vi "Write EEPROM User Area.vi"(8 "error in (no error)":errorcluster, 10 "User Area Data":u8[](array[numeric]) format="%x", 11 "Handle":u64) -> (0 "error out":errorcluster, 3 "Handle out":u64)   [LabVIEW 2019, in "D2XX-lv.lvlib"]
doc: "Write data into the EEPROM user area."
uses:
  D2XX-lv.lvlib
  <instrlib>/_D2XX/D2XX/D2XX.lvlib
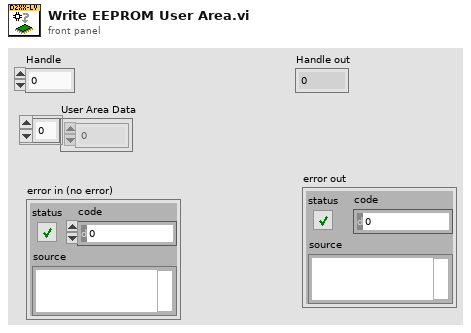
[diagram p1: front panel]
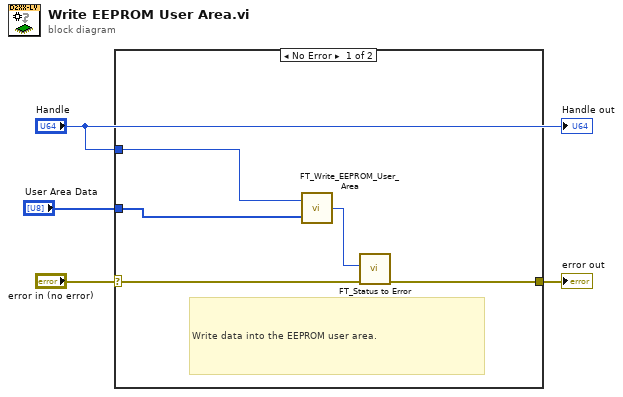
[diagram p0: block diagram]
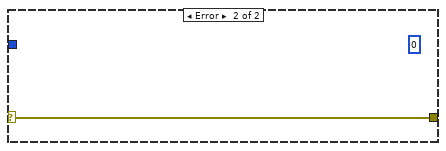
[diagram p2: hidden frame]
diagram:
  n1 = case shown="No Error" "error in (no error)" {
    selector: "error in (no error)" -> [w9 w10]
    tunnel: [w8 w10] -> w3
    tunnel: "Handle" -> [w6 _]
    tunnel: "User Area Data" -> [w5 _]
    frame No Error {
      # "Write data into the EEPROM user area."
      n2 = call <instrlib>:"FT_Write_EEPROM_User_Area.vi"("User Area Data In"=w5, "Handle"=w6) -> ("FT_Status"=w7:u32)
      n3 = call "FT_Status to Error.vi"("error in (no error)"=w9, "FT_Status"=w7) -> ("error out"=w8:errorcluster)  [unwired: 9 in]
    }
    frame Error {
      (unwired) u32 0 ("Bytes Written")
    }
  }
  "error out" <- w3
  "Handle out" <- "Handle"
